vi "Enqueue.vi"(6 "abort? (F)":bool, 7 "last element? (F)":bool, 8 "message":T2, 9 "event priority":T1=enum."normal priority", 10 "is valid? (T)":bool=TRUE, 11 "data in":refnum<class "EventMessengerPData.lvclass">) -> (0 "last element?":bool, 3 "data out":refnum<class "EventMessengerPData.lvclass">, 4 "aborted?":bool)   [LabVIEW 2020, in "Event Messenger Priority.lvlib" / "EventMessengerPData.lvclass"]
uses:
  EventMessengerPData.lvclass
  EventMessengerPData.lvclass/EventMessengerPData.ctl
  <vilib>/event_ctls.llb/usereventprio.ctl
  Element.ctl
  Event Messenger Priority.lvlib
  Event Data.ctl
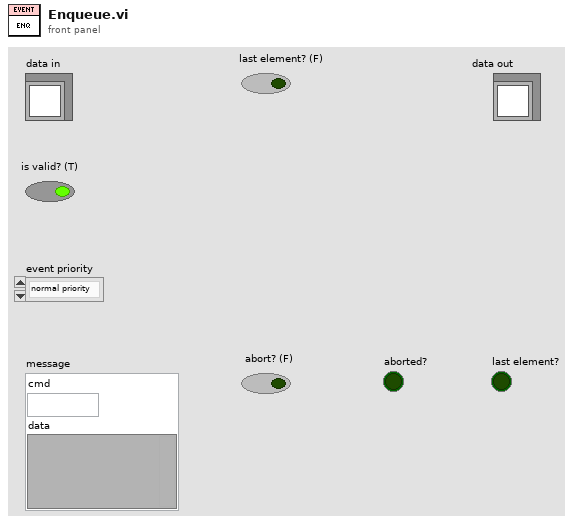
[diagram p1: front panel]
types:
  T1 = typedef "usereventprio.ctl" = enum32{"high priority", "normal priority"}
  T2 = typedef "Event Messenger Priority.lvlib/Element.ctl" = cluster{"cmd":string, "data":variant}
  T3 = typedef "Event Messenger Priority.lvlib/Event Data.ctl" = cluster{"message":T2, "msg valid?":bool, "last msg?":bool, "aborted?":bool, "priority?":bool}
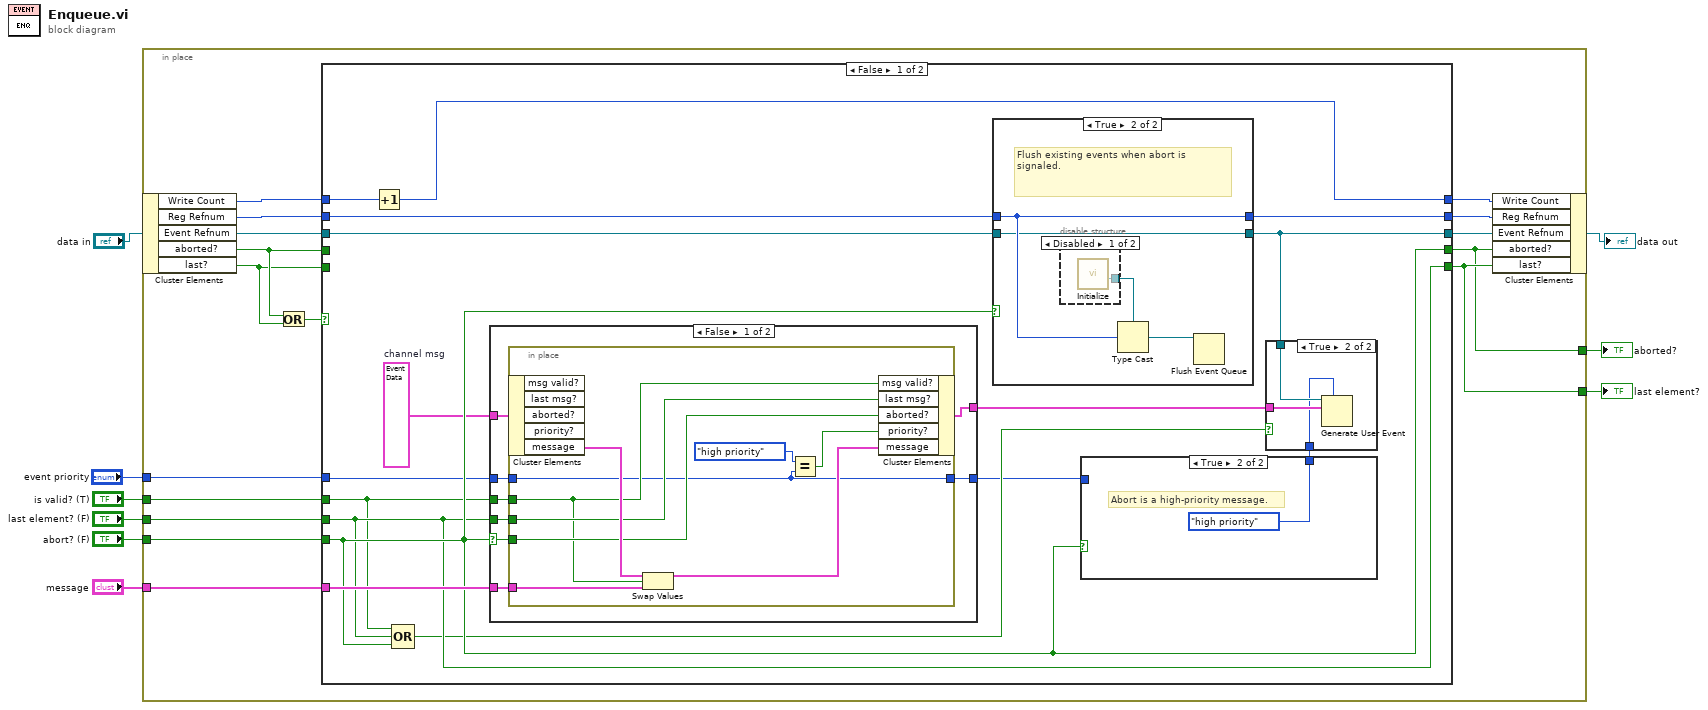
[diagram p0: block diagram]
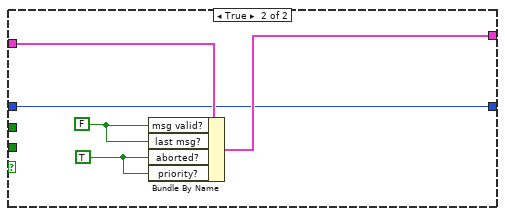
[diagram p2: hidden frame]
diagram:
  n1 = in-place {
    in-place-border: "message" -> [w23]
    in-place-border: "is valid? (T)" -> [w18]
    in-place-border: "last element? (F)" -> [w17]
    in-place-border: "abort? (F)" -> [w16]
    in-place-border: [w12] -> w3
    in-place-border: [w11] -> w2
    in-place-border: "event priority" -> [w10]
    n2 = in-place-cluster #1("data in") -> ("Write Count"=w25:u32, "Reg Refnum"=w19:u32, "Event Refnum"=w22:refnum<user-event>, "aborted?"=w14:bool, "last?"=w13:bool)
    n3 = Or(x=w14, y=w13) -> (x .or. y?=w15:bool)
    n4 = case shown="False" w15 {
      tunnel: w25 -> [w41 w80]
      tunnel: [w40 w80] -> w24
      tunnel: w23 -> [w38 _]
      tunnel: w22 -> [w35 w78]
      tunnel: [w36 w78] -> w21
      tunnel: [w34 w79] -> w20
      tunnel: w19 -> [w39 w79]
      tunnel: [w32 w77] -> w11
      tunnel: w18 -> [w30 _]
      tunnel: w17 -> [w31 _]
      tunnel: w16 -> [w32 _]
      tunnel: w14 -> [_ w77]
      tunnel: [w31 w76] -> w12
      tunnel: w13 -> [_ w76]
      tunnel: w10 -> [w28 _]
      frame False {
        w26 = T3 {"message"={"cmd"="", "data"=variant}, "msg valid?"=TRUE, "last msg?"=TRUE, "aborted?"=TRUE, "priority?"=FALSE}  # channel msg
        n5 = Increment(x=w41) -> (x+1=w40:u32)
        n6 = Compound Arithmetic op=OR(w30, w31, w32) -> (w29:bool)
        n7 = case shown="False" w32 {
          selector: w32 -> [w45 _]
          tunnel: w30 -> [w49 _]
          tunnel: w38 -> [w48 _]
          tunnel: [w47 w62] -> w37
          tunnel: w26 -> [w46 w63]
          tunnel: w31 -> [w44 _]
          tunnel: w28 -> [w43 w60]
          tunnel: [w42 w60] -> w27
          frame False {
            n8 = in-place {
              in-place-border: w49 -> [w53]
              in-place-border: w44 -> [w54]
              in-place-border: w45 -> [w55]
              in-place-border: w48 -> [w57]
              in-place-border: w43 -> [w50]
              in-place-border: [w50] -> w42
              n9 = in-place-cluster #2(w46) -> ("message"=w58:T2)  [unwired: 4 out]
              n10 = Swap Values(12:w58, 13:w53, 14:w57) -> (1:w56:T2)  [unwired: 1 out]
              n11 = Equal?(x=usereventprio."high priority" ("y"), y=w50) -> (x = y?=w51:bool)
              n12 = in-place-cluster #2("msg valid?"=w53, "last msg?"=w54, "aborted?"=w55, "priority?"=w51, "message"=w56) -> (w47:T3)
            }
          }
          frame True {
            w59 = TRUE ("last element?")
            w61 = FALSE ("element valid?")
            n13 = Bundle By Name(cluster=w63, "msg valid?"=w61, "last msg?"=w61, "aborted?"=w59, "priority?"=w59) -> (w62:T3)
          }
        }
        n14 = case shown="True" w32 {
          tunnel: [w70 w73] -> w36
          tunnel: w35 -> [w70 w73]
          tunnel: [w69 w74] -> w34
          tunnel: w39 -> [w69 w74]
          frame False {
            # "If not aborting, keep using the same refnum as previous Write calls."
          }
          frame True {
            # "Flush existing events when abort is signaled."
            n15 = disable-structure shown="Disabled" {
              disable-tunnel: [w75 _] -> w71
              frame Disabled {
                n16 = call "Initialize.vi"() -> ("Event Registration Refnum"=w75:refnum<event-registration>)  [unwired: 10 in, 1 out]
              }
              frame Enabled {
              }
            }
            n17 = Type Cast(type=w71, x=w74) -> (*(type *) &x=w72:refnum<event-registration>)
            n18 = Flush Event Queue(0:w72) -> ()  [unwired: 5 in, 3 out]
          }
        }
        n19 = case shown="True" w32 {
          tunnel: w27 -> [w67 _]
          tunnel: [w67 usereventprio."high priority" ("event priority")] -> w33
          frame False {
          }
          frame True {
            # "Abort is a high-priority message."
          }
        }
        n20 = case shown="True" w29 {
          tunnel: w37 -> [_ w66]
          tunnel: w36 -> [_ w65]
          tunnel: w33 -> [_ w64]
          frame False {
          }
          frame True {
            n21 = Generate User Event(priority (normal)=w64, user event=w65, event data cluster=w66) -> ()  [unwired: 1 in, 2 out]
          }
        }
      }
      frame True {
        # "If aborted or last element has already been sent on previous writes then this channel is done until it gets re-initialized, so don't do anything now."
      }
    }
    n22 = in-place-cluster #1("Write Count"=w24, "Reg Refnum"=w20, "Event Refnum"=w21, "aborted?"=w11, "last?"=w12) -> (→"data out":refnum<class "EventMessengerPData.lvclass">)
  }
  "aborted?" <- w2
  "last element?" <- w3
